vi "Flag_Write.vi"(8 "error in (no error)":errorcluster, 11 "Flag":T1) -> (0 "error out":errorcluster)   [LabVIEW 2016, in "SeqProcessor.lvlib"]
uses:
  SeqProcessor.lvlib
  controls/Flag.ctl
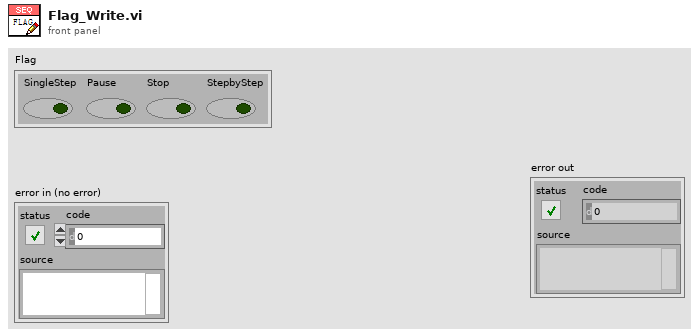
[diagram p1: front panel]
types:
  T1 = typedef "SeqProcessor.lvlib/Flag.ctl" = cluster{"SingleStep":bool, "Pause":bool, "Stop":bool, "StepbyStep":bool}
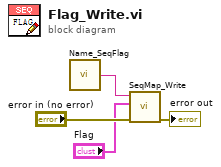
[diagram p0: block diagram]
diagram:
  n1 = call "Name_SeqFlag.vi"() -> ("SeqFlag"=w1:string)  [unwired: 5 in]
  n2 = call "SeqMap_Write.vi"("error in (no error)"="error in (no error)", "Value"="Flag", "Tag"=w1) -> ("error out"=→"error out":errorcluster)  [unwired: 8 in]
